vi "Apply Endpoint Configuration.vi"(8 "error in":errorcluster, 9 "endpoint":string, 10 "endpoint configuration in":T2 format="%.0x", 11 "slsc switch session in":T1) -> (0 "error out":errorcluster, 1 "endpoint addressable?":bool, 2 "endpoint configuration out":T2 format="%.0x", 3 "slsc switch session out":T1)   [LabVIEW 2017, in "NI-SWITCH Scripting.lvlib"]
uses:
  NI-SWITCH Scripting.lvlib
  <vilib>/NI Veristand/Custom Device API/Custom Device Item Ref.ctl
  <vilib>/userdefined/High Color/SLSC_Switch/nislscslSession.ctl
  <resource>/objmgr/nislscsl.rc
  <vilib>/NI VeriStand/Custom Device API/Custom Device API.lvlib
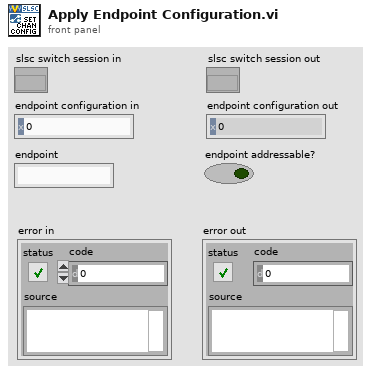
[diagram p1: front panel]
types:
  T1 = typedef "nislscslSession.ctl" = refnum<k20>
  T2 = typedef "Custom Device API.lvlib/Custom Device Item Ref.ctl" = u64
  T3 = typedef "NI-SWITCH Shared.lvlib/Endpoint Configuration Enum.ctl" = enum16{"Load", "Source", "Configuration"}
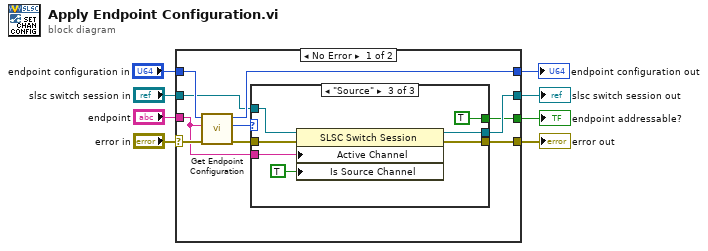
[diagram p0: block diagram]
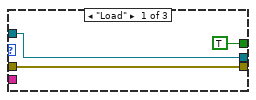
[diagram p2: hidden frame]
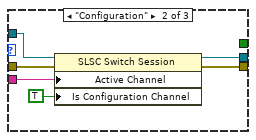
[diagram p3: hidden frame]
diagram:
  n1 = case shown="No Error" "error in" {
    selector: "error in" -> [w14 w37]
    tunnel: [w18 w35] -> w8
    tunnel: [w17 w37] -> w7
    tunnel: [w15 w36] -> w6
    tunnel: "endpoint configuration in" -> [w13 w35]
    tunnel: "endpoint" -> [w12 _]
    tunnel: [w10 _] -> w2
    tunnel: "slsc switch session in" -> [w9 w36]
    frame No Error {
      n2 = call "Get Endpoint Configuration.vi"("error in"=w14, "endpoint"=w12, "endpoint configuration in"=w13) -> ("error out"=w16:errorcluster, "configuration"=w11:T3, "endpoint configuration out"=w18:T2)  [unwired: 6 in]
      n3 = case shown="\"Source\"" w11 {
        tunnel: w9 -> [w20 w26 w34]
        tunnel: w12 -> [_ w27 w32]
        tunnel: [TRUE _ TRUE] -> w10
        tunnel: [w20 w24 w30] -> w15
        tunnel: w16 -> [w19 w23 w28]
        tunnel: [w19 w22 w29] -> w17
        frame "Load" {
        }
        frame "Configuration" {
          n4 = property class="SLSC Switch Session"(reference=w26, error in=w23, "Active Channel"=w27, "Is Configuration Channel"=TRUE ("Channel Configuration:Is Configuration Channel")) -> (reference out=w24:T1, error out=w22:errorcluster)
        }
        frame "Source" {
          n5 = property class="SLSC Switch Session"(reference=w34, error in=w28, "Active Channel"=w32, "Is Source Channel"=TRUE ("Channel Configuration:Is Source Channel")) -> (reference out=w30:T1, error out=w29:errorcluster)
        }
      }
    }
    frame Error {
    }
  }
  "endpoint configuration out" <- w8
  "error out" <- w7
  "slsc switch session out" <- w6
  "endpoint addressable?" <- w2
